vi "rpr -- view segment files.vi"(10 "segment index":i32=2, 11 "9w folder path":path=path "C:/data/RUS/Experiment/ProbeTest/Probe10/YBCO_5/sweep2/9w") -> (0 "Array":dbl[][](array[numeric]), 2 "temperature points OUT":dbl[](array[numeric])=[12.04, 12.515, 12.958, 13.385, 13.835, 14.277, 15.156, 15.602, 16.045, 16.487, 16.932, 17.359, 17.798, 18.261, 19.127, 19.573, 20.016, 20.451, 20.896, 21.339, 21.788, 22.231, 22.667, 23.119, 23.569, 24.031, 24.481, 24.933, 25.403, 25.864, 26.33, 26.779, 27.724, 28.2, 28.669, 29.151, 29.63, 30.11, 30.597, 31.071, 31.547, 32.039, 32.526, 33.027, 33.522, 34.022, 34.517, 36.984, 37.471, 37.971, 38.467, 38.955, 39.451, 39.952, 40.442, 40.944, 41.448, 41.947, 42.45, 42.941, 43.431, 43.924, 44.432, 45.431, 45.929, 46.433, 46.939, 47.435, 47.929, 48.425, 48.917, 49.41, 49.914, 50.413, 50.911, 51.907, 52.399, 52.895, 53.388, 53.886, 54.386, 54.88, 55.878, 56.37, 57.351, 57.838, 58.333, 58.83, 59.327, 60.304, 60.797, 61.288, 61.778, 62.268, 62.758, 63.251, 63.742, 64.228, 64.713, 65.207, 65.703, 66.192, 66.68, 67.166, 67.653, 68.147, 68.637, 69.126, 69.613, 70.1, 70.591, 71.079, 71.57, 72.054, 72.541, 73.024, 73.521, 74.008, 74.5, 74.988, 75.475, 75.96, 76.449, 76.94, 77.431, 77.921, 78.414, 78.908, 79.395, 79.884, 80.373, 80.865, 81.356, 81.846, 82.329, 82.821, 83.31, 83.795, 84.288, 84.777, 85.27, 85.759, 86.249, 86.739, 87.233, 87.72, 88.214, 88.704, 89.201, 89.692, 90.181, 90.668, 91.464, 91.954, 92.445, 92.929, 93.425, 93.91, 94.401, 94.89, 95.378, 95.865, 96.359, 96.847, 97.332, 97.82, 98.312, 98.797, 99.289, 99.779, 100.268, 100.757, 101.249, 101.738, 102.226, 102.72, 103.205, 103.692, 104.18, 104.672, 105.154, 105.643, 106.124, 106.612, 107.103, 107.589, 108.144, 108.635, 109.126, 109.613, 110.102, 110.593, 111.09, 111.592, 112.103, 112.591, 113.076, 113.558, 114.039, 114.522, 115.001, 115.483, 115.967, 116.445, 116.923, 117.404, 117.884, 118.365, 118.852, 119.336, 119.826, 120.314, 120.802, 121.289, 121.781, 122.269, 122.759, 123.251, 123.74, 124.223, 124.717, 125.21, 125.701, 126.19, 126.684, 127.175, 127.666, 128.152, 128.648, 129.137, 129.629, 130.119, 130.61, 131.101, 131.591, 132.086, 132.578, 133.073, 133.56, 134.054, 134.538, 135.03, 135.522, 136.018, 136.506, 136.995, 137.484, 137.974, 138.463, 138.956, 139.45, 139.943, 140.435, 140.921, 141.413, 141.91, 142.403, 142.896, 143.394, 143.884, 144.378, 144.875, 145.367, 145.86, 146.351, 146.846, 147.334, 147.83, 148.318, 148.811, 149.302, 149.793, 150.285, 150.78, 151.271, 151.763, 152.263, 152.756, 153.247, 153.737, 154.228, 154.726, 155.225, 155.713, 156.208, 156.7, 157.188, 157.682, 158.173, 158.665, 159.155, 159.65, 160.136, 160.631, 161.123, 161.624, 162.2, 162.724, 163.084, 163.519, 164.002, 164.5, 165.01, 165.511, 166.014, 166.512, 167.008, 167.502, 167.995, 168.985, 169.477, 170.461, 170.955, 171.446, 171.93, 172.427, 172.921, 173.425, 173.92, 174.414, 175.404, 175.898, 176.391, 176.89, 177.385, 177.878, 178.366, 178.862, 179.352, 179.851, 180.348, 180.838, 181.329, 181.823, 182.317, 182.815, 183.309, 183.802, 184.3, 184.794, 185.288, 185.78, 186.279, 186.772, 187.266, 187.763, 188.26, 188.757, 189.249, 189.744, 190.238, 190.728, 191.216, 191.714, 192.21, 192.697, 193.191, 193.678, 194.177, 194.672, 195.171, 195.66, 196.158, 196.649, 197.146, 197.638, 198.134, 198.629, 199.125, 199.617, 200.108, 200.601, 201.091, 201.58, 202.071, 203.059, 203.546, 204.037, 204.531, 205.022, 205.518, 206.009, 206.501, 206.996, 207.48, 207.974, 208.465, 208.959, 209.452, 209.947, 210.438, 210.926, 211.42, 211.913, 212.404, 212.897, 213.391, 213.876, 214.374, 214.865, 215.358, 215.85, 216.34, 216.838, 217.331, 217.829, 218.32, 218.814, 219.313, 219.801, 220.295, 220.786, 221.287, 221.782, 222.284, 222.781, 223.279, 223.779, 224.273, 224.779, 225.304, 225.778, 226.237, 226.715, 227.217, 227.722, 228.224, 228.724, 229.213, 229.709, 230.21, 230.703, 231.195, 231.691, 232.18, 232.676, 233.165, 233.667, 234.156, 234.651, 235.146, 235.643, 236.134, 236.633, 237.128, 237.622, 238.113, 238.614, 239.113, 239.612, 240.108, 240.599, 241.095, 241.59, 242.087, 242.588, 243.091, 243.586, 244.085, 244.586, 245.078, 245.58, 246.073, 246.568, 247.064, 247.566, 248.068, 248.568, 249.064, 249.563, 250.064, 250.558, 251.052, 251.55, 252.061, 252.549, 253.048, 253.546, 254.049, 254.544, 255.032, 255.529, 256.016, 256.507, 257.007, 257.507, 257.999, 258.493, 258.992, 259.486, 259.984, 260.477, 260.973, 261.47, 261.97, 262.475, 262.97, 263.467, 263.966, 264.468, 264.961, 265.469, 265.966, 266.458, 266.956, 267.461, 267.942, 268.433, 268.936, 269.434, 269.923, 270.424, 270.908, 271.399, 271.896, 272.392, 272.876, 273.383, 273.861, 274.358, 274.85, 275.341, 275.836, 276.322, 276.824, 277.316, 277.809, 278.305, 278.805, 279.312, 279.794, 280.295, 280.787, 281.284, 281.793, 282.287, 282.779, 283.278, 283.778, 284.276, 284.779, 285.28, 285.773, 286.28, 286.775, 287.278, 287.769, 288.266, 288.765, 289.256, 289.761, 290.255, 290.76, 291.261, 291.755, 292.257, 292.749, 293.243, 293.746, 294.245, 294.74, 295.236, 295.732, 296.225, 296.72, 297.201, 297.713, 298.202, 298.691, 299.189, 299.653, 299.79], 3 "peaks":i32[](array[numeric])=[556, 646, 974, 1127, 1578, 1759, 1872, 1895, 2216, 2256, 2345], 4 "# of temperatures":i32, 6 "# of peaks":i32)   [LabVIEW 2010]
panel:
  in  "what":T1(ring)
  out "all peaks":i32[](array[numeric])=[556, 646, 974, 1127, 1207, 1578, 1759, 1872, 1895, 2004, 2216, 2256, 2345]
  in  "buttons":bool[](array[boolean])=[TRUE, TRUE, TRUE, TRUE, FALSE, TRUE, TRUE, TRUE, TRUE, FALSE, TRUE, TRUE, TRUE, TRUE, TRUE, TRUE, TRUE, TRUE, TRUE, TRUE]
  out "Plot:   elastic vs temp 2":cluster{dbl[], dbl[]}[](graph)
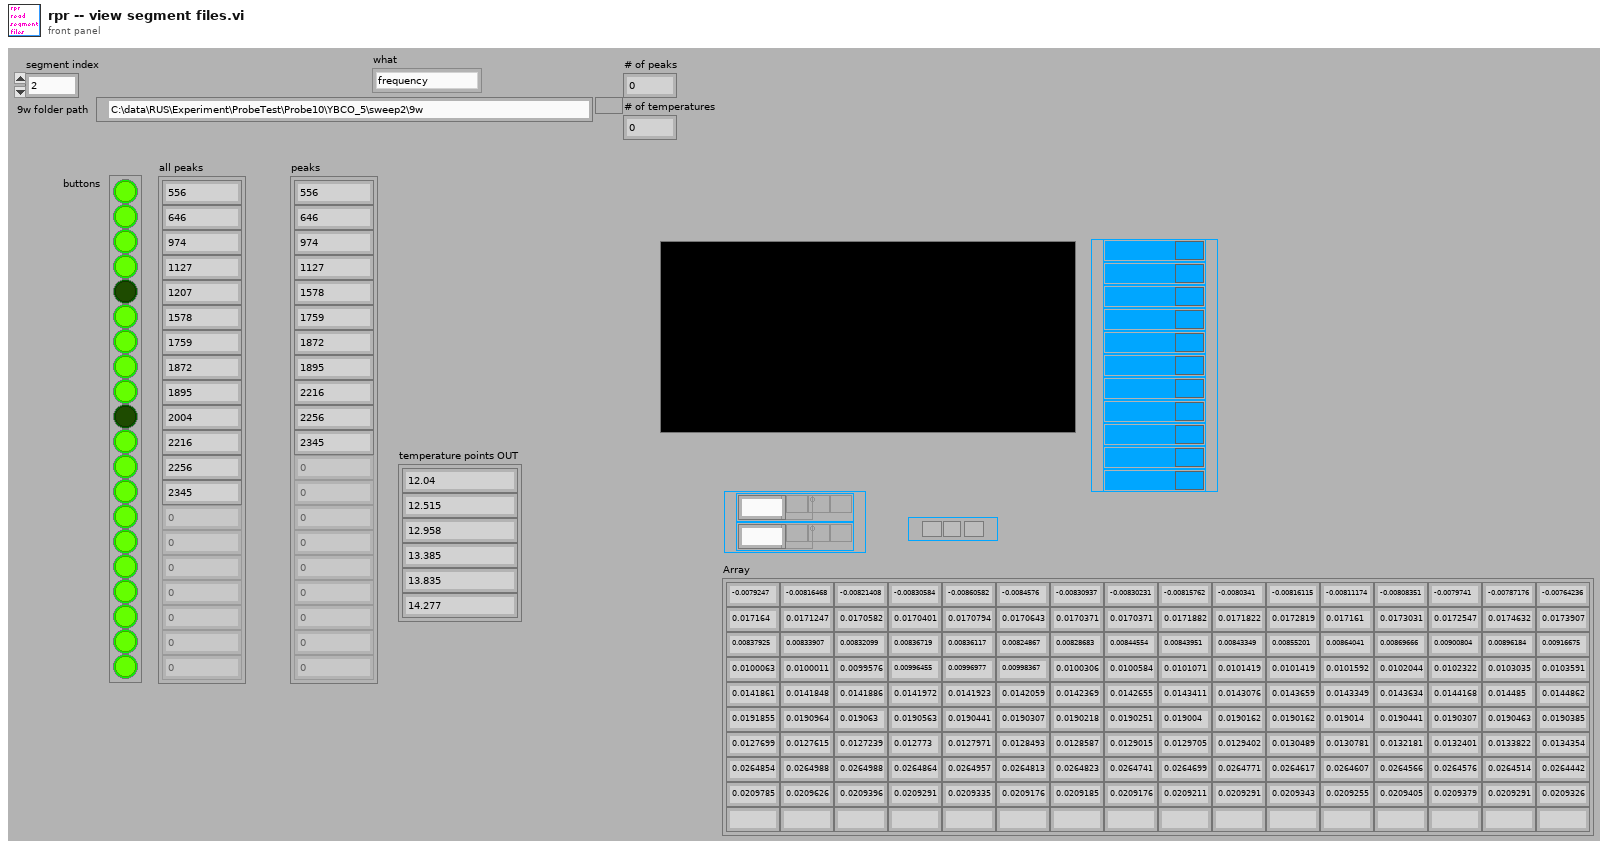
[diagram p1: front panel]
types:
  T1 = enum16{"frequency", "attenuation", "deltafreq", "Vardeltafreq"}
  T2 = cluster{"temperature points OUT":dbl[], "Array":dbl[]}
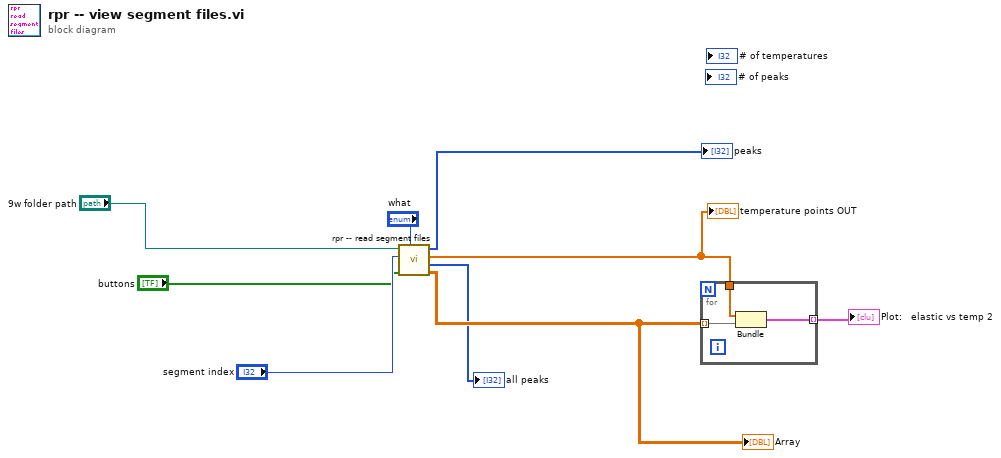
[diagram p0: block diagram]
diagram:
  n1 = call "rpr -- read segment files.vi"("what"="what", "buttons"="buttons", "segment index"="segment index", "9w folder path"="9w folder path") -> ("Array"=w4:dbl[][], "all peaks"=→"all peaks":i32[], "temperature points OUT"=w6:dbl[], "peaks"=→"peaks":i32[])  [unwired: 2 in, 2 out]
  "Array" <- w4
  "temperature points OUT" <- w6
  n2 = for {
    tunnel: [w12] -> w5 mode=indexing
    tunnel: w4 -> [w11] mode=indexing
    tunnel: w6 -> [w10]
    n3 = Bundle("temperature points OUT"=w10, "Array"=w11) -> (w12:T2)  [unwired: 1 in]
  }
  "Plot:   elastic vs temp 2" <- w5
